vi "Send Operation Complete Msg.vi"(8 "error in":errorcluster, 10 "Operation Complete":bool, 11 "Generic Optimization in":refnum<class "Generic Optimization.lvclass">) -> (0 "error out":errorcluster, 3 "Generic Optimization out":refnum<class "Generic Optimization.lvclass">)   [LabVIEW 2018, in "Generic Optimization Actor.lvlib" / "Generic Optimization.lvclass"]
uses:
  Generic Optimization.lvclass
  C:/Program Files (x86)/National Instruments/LabVIEW 2018/vi.lib/ActorFramework/Actor/Actor.lvclass
  <vilib>/ActorFramework/Actor/Actor.lvclass/Actor.ctl
  Generic Optimization.lvclass/Generic Optimization.ctl
  Generic Optimization Messages/Operation Complete Msg/Operation Complete Msg.lvclass/Operation Complete Msg.ctl
  <vilib>/ActorFramework/Message Enqueuer/Message Enqueuer.lvclass/Message Enqueuer.ctl
  <vilib>/ActorFramework/Message Enqueuer/Enqueue.vi
  Generic Optimization Messages/Operation Complete Msg/Operation Complete Msg.lvclass
  C:/Program Files (x86)/National Instruments/LabVIEW 2018/vi.lib/ActorFramework/Message/Message.lvclass
  <vilib>/ActorFramework/Message Priority Queue/Priority Enqueue.vi
  <vilib>/ActorFramework/Actor/Actor.lvclass
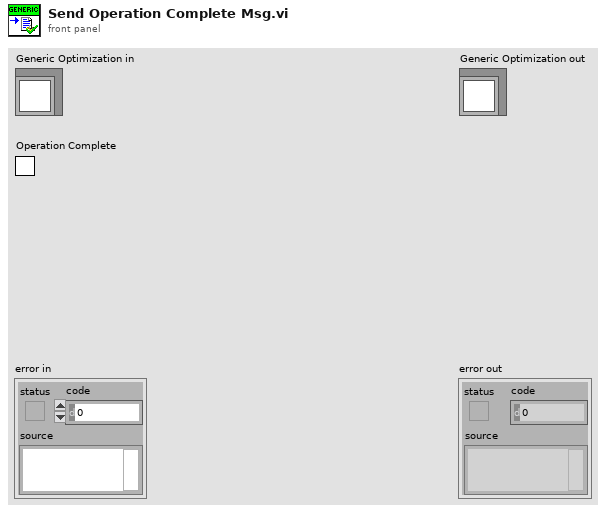
[diagram p1: front panel]
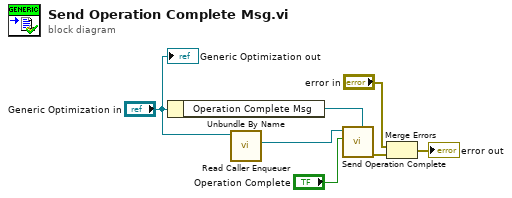
[diagram p0: block diagram]
diagram:
  n1 = Unbundle By Name("Generic Optimization in") -> ("Operation Complete Msg"=w5:refnum<class "Operation Complete Msg.lvclass">)
  n2 = call <vilib>:"Read Caller Enqueuer.vi"("Actor"="Generic Optimization in") -> ("Caller Enqueuer"=w4:refnum<class "Message Enqueuer.lvclass">)  [unwired: 10 in]
  n3 = call "Send Operation Complete.vi"("Operation Complete Msg"=w5, "Operation Complete"="Operation Complete", "Message Enqueuer in"=w4) -> ("error out"=w2:errorcluster)  [unwired: 7 in, 1 out]
  n4 = Merge Errors("error in", w2) -> (→"error out":errorcluster)
  "Generic Optimization out" <- "Generic Optimization in"
